vi "Main_v2.vi"() -> ()   [LabVIEW 2018]
uses:
  <userlib>/Gigahertz-Optik/GOMDTR9600/GOMDTR9600.lvlib
panel:
  out "Pulse Begin (ms)":dbl format="%.4f"
  out "Pulse End (ms)":dbl format="%.4f"
  out "Maximum Pulse":cluster{i32[], dbl[]}(graph) caption="Spectrum"
  out "Pulse_Time (µs)":dbl format="%.2f"
  out "Pulse_Energy (V/s)":dbl
  in  "Resolution":u32=10000000
  in  "range100ns":string(combo) caption="Range"
  out "Serial":string
  in  "Sampling Rate":T1(radio)
  in  "range1us":string(combo)="2" caption="Range"
  out "Progress":i32
  in  "ReleaseHandle":bool
  out "Single Measurement":cluster{dbl[], dbl[]}(graph) caption="Spectrum"
  out "State":i32
  in  "measure":bool
  out "Status":string
  # "PULSE ENERGY ANALYZER"
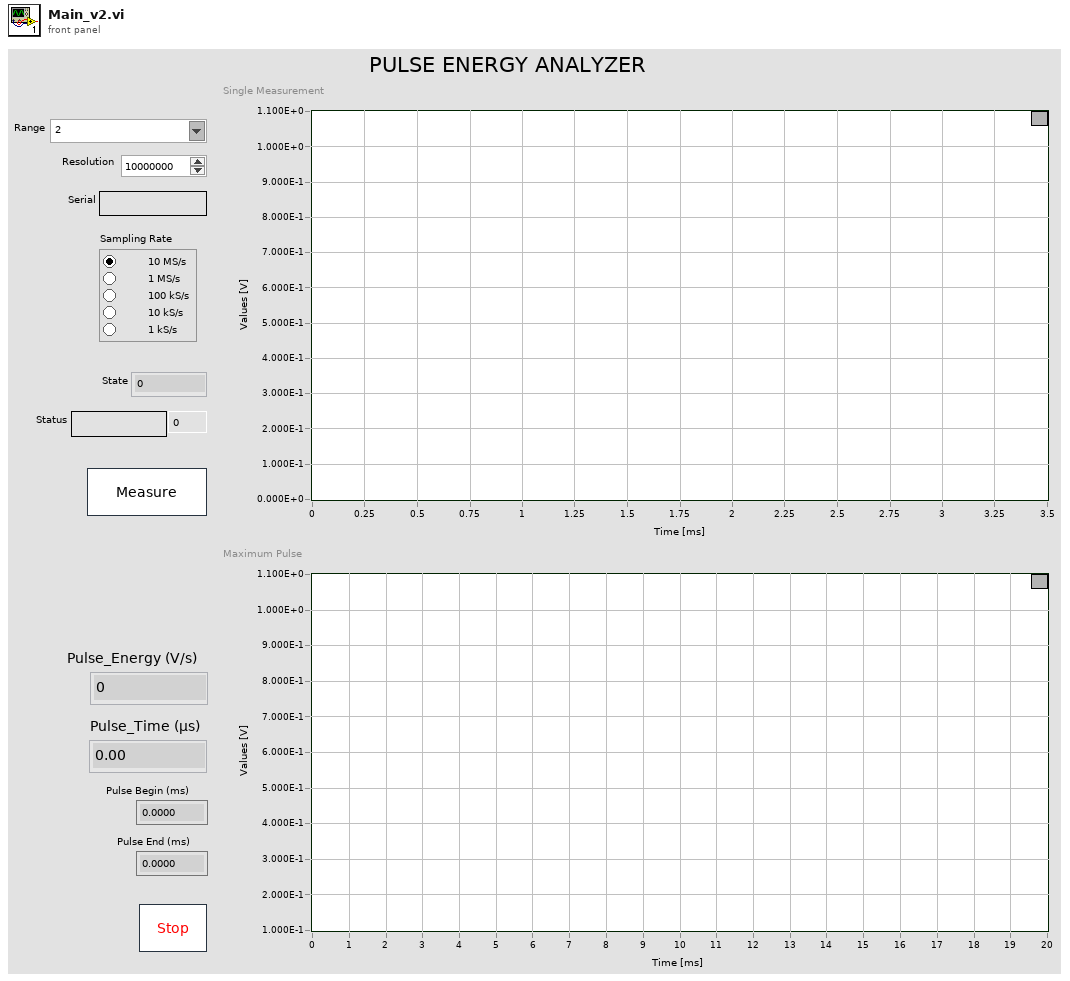
[diagram p1: front panel]
types:
  T1 = enum32{"10MS/s", "1MS/s", "100kS/s", "10kS/s", "1kS/s"}
  T2 = cluster{"address":i32, "mean value":dbl, "min value":dbl, "max value":dbl}[][]
  T3 = enum32{"invalid app kind", "Development System", "Run Time System", "Student Edition", "Embedded LabVIEW", "Evaluation", "Custom"}
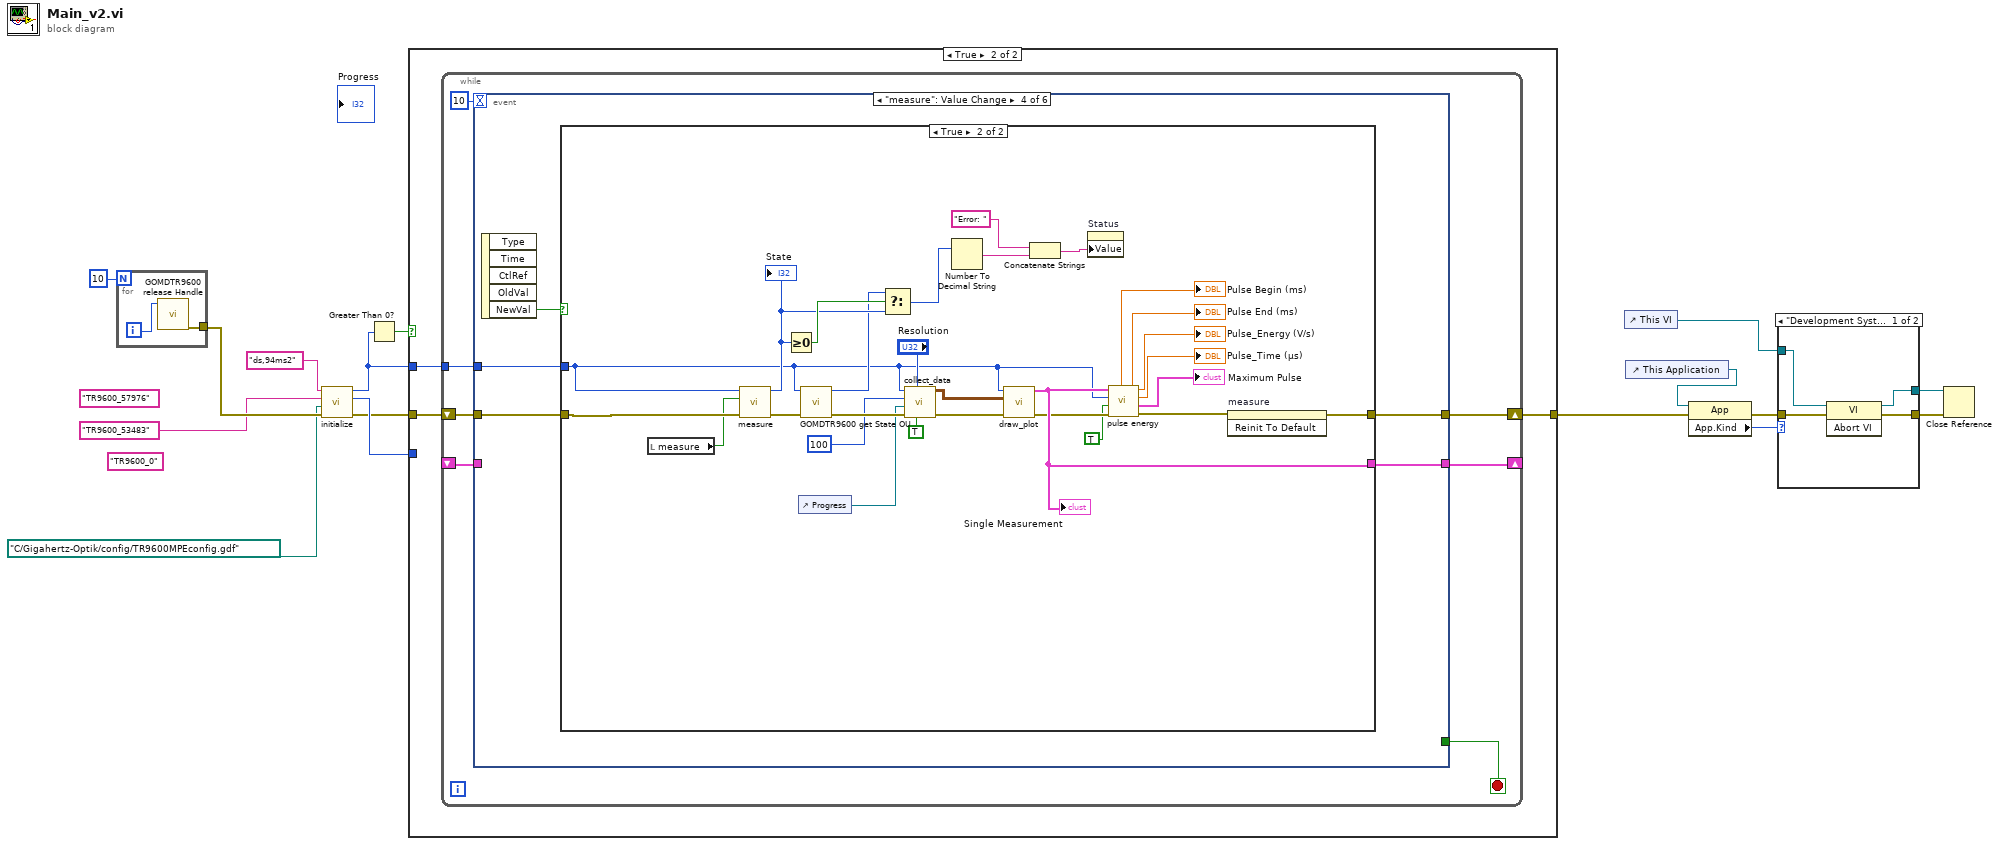
[diagram p0: block diagram]
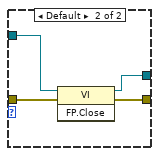
[diagram p2: hidden frame]
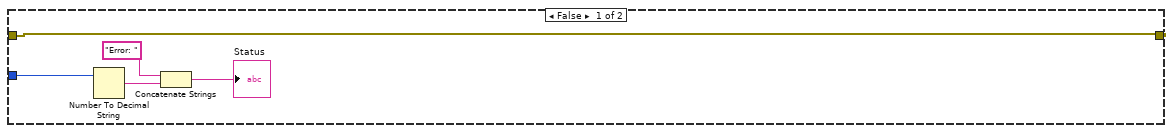
[diagram p3: hidden frame]
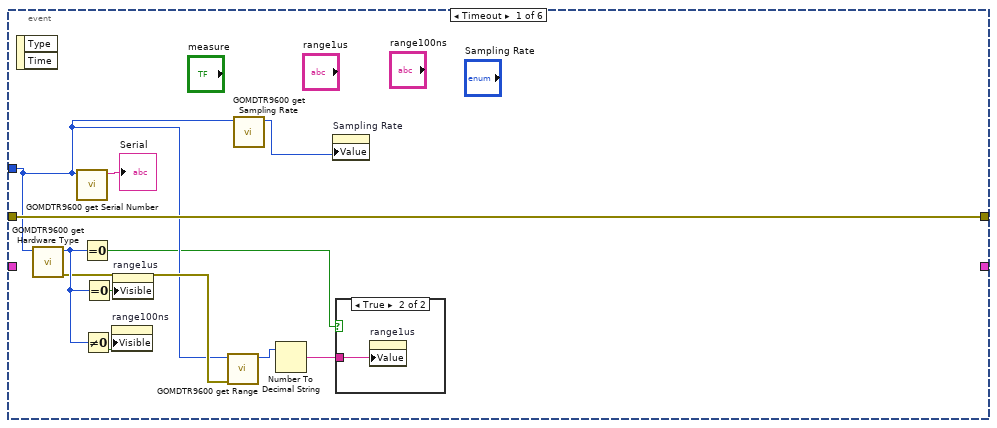
[diagram p4: hidden frame]
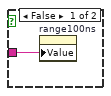
[diagram p5: hidden frame]
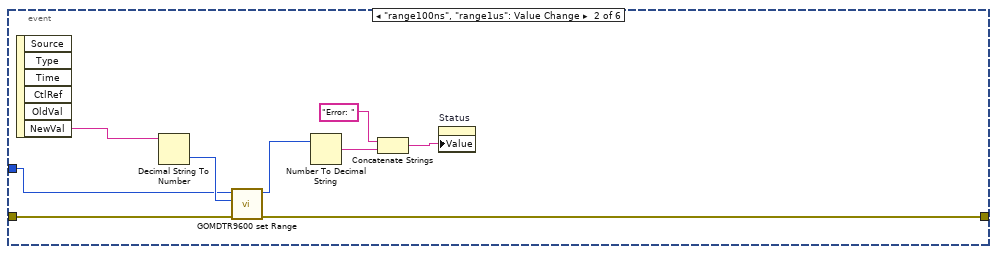
[diagram p6: hidden frame]
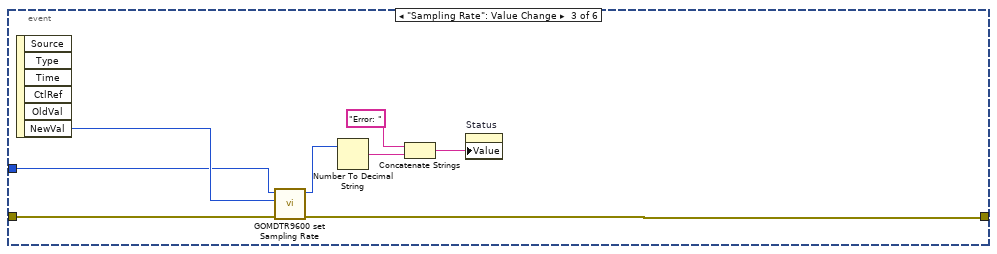
[diagram p7: hidden frame]
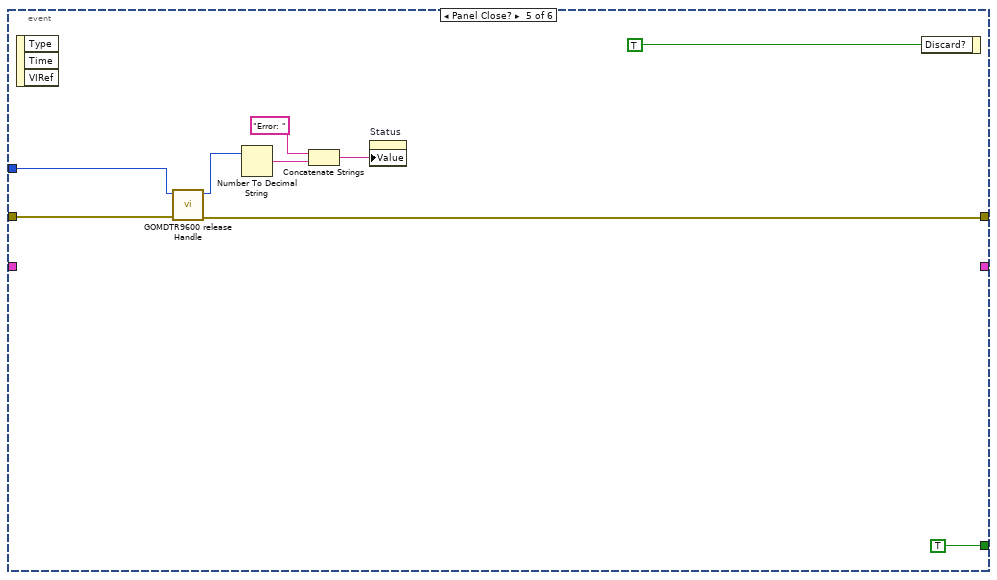
[diagram p9: hidden frame]
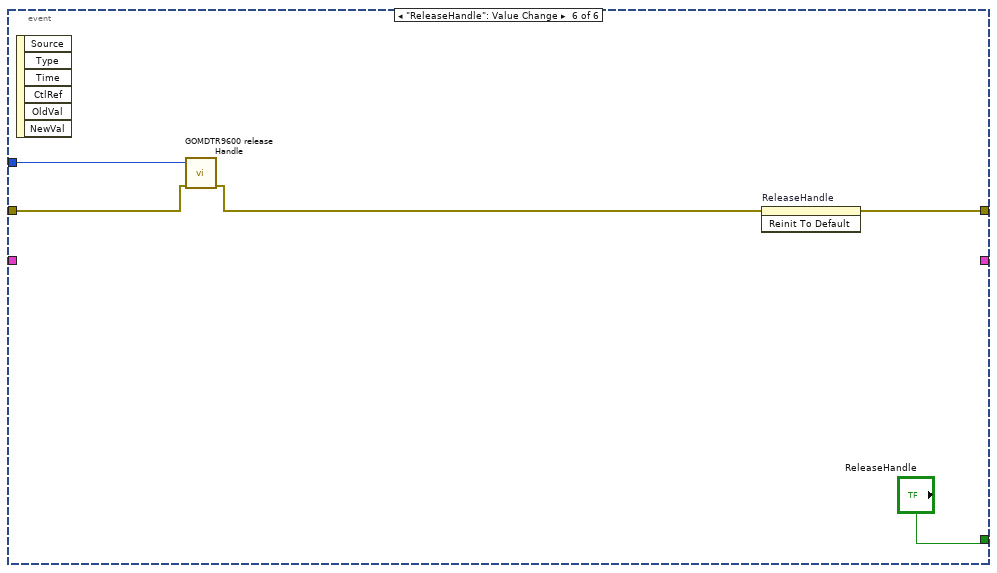
[diagram p10: hidden frame]
diagram:
  (unwired) "TR9600_57976" ("deviceName")
  (unwired) "TR9600_0" ("deviceName")
  n1 = for {
    N: 10 -> [_]
    tunnel: [w17] -> w4
    i -> [w18]
    n2 = call <userlib>:"GOMDTR9600 release Handle.vi"("handle"=w18) -> ("error out"=w17:errorcluster)  [unwired: 9 in, 1 out]
  }
  n3 = call "initialize.vi"("error in (no error)"=w4, "Optometer cfg file"=path "C:/Gigahertz-Optik/config/TR9600MPEconfig.gdf" ("filename"), "deviceName"="TR9600_53483", "password"="ds,94ms2") -> ("error out"=w6:errorcluster, "function return"=w7:i32, "handle"=w3:i32)  [unwired: 5 in]
  n4 = Greater Than 0?(x=w3) -> (x > 0?=w16:bool)
  n5 = case shown="True" w16 {
    tunnel: w3 -> [_ w25]
    tunnel: w6 -> [w19 w26]
    tunnel: w7 -> [w23 _]
    tunnel: [w19 w24] -> w10
    frame False {
      n6 = Number To Decimal String(number=w23) -> (decimal integer string=w21:string)  [unwired: 1 in]
      n7 = Concatenate Strings("Error: ", w21) -> (→"Status":string)
    }
    frame True {
      n8 = while {
        shift-right: [w31] -> w24
        shift-left: w26 -> [w33]
        tunnel: w25 -> [w32]
        shift-right: [w28] -> _
        shift-left: _ -> [w27]
        stop <- w30 stop-if-true
        n9 = event shown="[3] \"measure\": Value Change" {
          selector: _ -> [_ _ _ _ _ _]
          dyn-events: _ -> [_ _ _ _ _ _]
          timeout: 10 -> [_ _ _ _ _ _]
          tunnel: w33 -> [w44 w48 w57 w67 w106 w110]
          tunnel: w32 -> [w35 w49 w58 w66 w105 w111]
          tunnel: [w44 w47 w56 w68 w104 w107] -> w31
          tunnel: [_ _ _ _ TRUE "ReleaseHandle"] -> w30
          tunnel: [_ _ _ w64 _ _] -> w28
          tunnel: w27 -> [_ _ _ _ _ _]
          event Timeout {
            n10 = event-data() -> ()  [unwired: 1 in, 2 out]
            n11 = call <userlib>:"GOMDTR9600 get Hardware Type.vi"("handle"=w35) -> ("error out"=w36:errorcluster, "value"=w39:i32)  [unwired: 8 in, 1 out]
            n12 = call <userlib>:"GOMDTR9600 get Serial Number.vi"("handle"=w35) -> ("value"=→"Serial":string)  [unwired: 8 in, 2 out]
            n13 = Equal To 0?(x=w39) -> (x = 0?=w34:bool)
            n14 = Not Equal To 0?(x=w39) -> (x != 0?=w37:bool)
            n15 = Equal To 0?(x=w39) -> (x = 0?=w38:bool)
            n16 = property on="range100ns" class="CmbBox"("Visible"=w37) -> ()  [unwired: 2 in, 2 out]
            n17 = property on="range1us" class="CmbBox"("Visible"=w38) -> ()  [unwired: 2 in, 2 out]
            n18 = call <userlib>:"GOMDTR9600 get Range.vi"("error in (no error)"=w36, "handle"=w35) -> ("value"=w40:i32)  [unwired: 7 in, 2 out]
            n19 = call <userlib>:"GOMDTR9600 get Sampling Rate.vi"("handle"=w35) -> ("value"=w42:i32)  [unwired: 8 in, 2 out]
            n20 = Number To Decimal String(number=w40) -> (decimal integer string=w41:string)  [unwired: 1 in]
            n21 = property on="Sampling Rate" class="RadioBtnsControl (strict)"("Value"=w42) -> ()  [unwired: 2 in, 2 out]
            n22 = case shown="True" w34 {
              tunnel: w41 -> [w45 w46]
              frame False {
                n23 = property on="range100ns" class="CmbBox"("Value"=w45) -> ()  [unwired: 2 in, 2 out]
              }
              frame True {
                n24 = property on="range1us" class="CmbBox"("Value"=w46) -> ()  [unwired: 2 in, 2 out]
              }
            }
          }
          event "range100ns", "range1us": Value Change {
            n25 = event-data() -> ("NewVal"=w50:string)  [unwired: 1 in, 5 out]
            n26 = Decimal String To Number(string=w50) -> (number=w55:i32)  [unwired: 2 in, 1 out]
            n27 = call <userlib>:"GOMDTR9600 set Range.vi"("error in (no error)"=w48, "value"=w55, "handle"=w49) -> ("error out"=w47:errorcluster, "function return"=w51:i32)  [unwired: 7 in]
            n28 = Number To Decimal String(number=w51) -> (decimal integer string=w52:string)  [unwired: 1 in]
            n29 = Concatenate Strings("Error: ", w52) -> (w54:string)
            n30 = property on="Status" class="Str"("Value"=w54) -> ()  [unwired: 2 in, 2 out]
          }
          event "Sampling Rate": Value Change {
            n31 = event-data() -> ("NewVal"=w59:T1)  [unwired: 1 in, 5 out]
            n32 = call <userlib>:"GOMDTR9600 set Sampling Rate.vi"("error in (no error)"=w57, "value"=w59, "handle"=w58) -> ("error out"=w56:errorcluster, "function return"=w60:i32)  [unwired: 7 in]
            n33 = Number To Decimal String(number=w60) -> (decimal integer string=w61:string)  [unwired: 1 in]
            n34 = Concatenate Strings("Error: ", w61) -> (w63:string)
            n35 = property on="Status" class="Str"("Value"=w63) -> ()  [unwired: 2 in, 2 out]
          }
          event "measure": Value Change {
            n36 = event-data() -> ("NewVal"=w65:bool)  [unwired: 1 in, 4 out]
            n37 = case shown="True" w65 {
              tunnel: [w69 w97] -> w68
              tunnel: w67 -> [w69 w86]
              tunnel: w66 -> [_ w72]
              tunnel: [_ w76] -> w64
              frame False {
              }
              frame True {
                n38 = local read "measure"() -> (w83:bool)
                n39 = call "measure.vi"("error in (no error)"=w86, "Measure"=w83, "handle"=w72) -> ("error out"=w92:errorcluster, "state"=w89:i32)  [unwired: 7 in]
                "State" <- w89
                n40 = Greater Or Equal To 0?(x=w89) -> (x >= 0?=w90:bool)
                n41 = control-ref of="Progress"() -> (w85:refnum<vi>)
                n42 = call <userlib>:"GOMDTR9600 get State OU.vi"("error in (no error)"=w92, "handle"=w72) -> ("error out"=w91:errorcluster, "value"=w88:i32)  [unwired: 7 in, 1 out]
                n43 = Select(t=w88, s=w90, f=w89) -> (s? t:f=w87:i32)
                n44 = call "collect_data.vi"("data?"=TRUE, "Resolution"="Resolution", "error in (no error)"=w91, "progress"=w85, "No. of values"=100, "handle"=w72) -> ("error out"=w96:errorcluster, "Dataset"=w80:T2)  [unwired: 4 in]
                n45 = Number To Decimal String(number=w87) -> (decimal integer string=w93:string)  [unwired: 1 in]
                n46 = call "draw_plot.vi"("error in (no error)"=w96, "Dataset"=w80, "handle"=w72) -> ("error out"=w74:errorcluster, "Plot"=w76:cluster{dbl[], dbl[]})  [unwired: 7 in]
                "Single Measurement" <- w76
                n47 = Concatenate Strings("Error: ", w93) -> (w95:string)
                n48 = property on="Status" class="Str"("Value"=w95) -> ()  [unwired: 2 in, 2 out]
                n49 = call "pulse energy.vi"("error in (no error)"=w74, "Boolean"=TRUE, "handle"=w72, "Spectrum"=w76) -> ("error out"=w75:errorcluster, "MaxPulse"=→"Maximum Pulse":cluster{i32[], dbl[]}, "Pulse_time"=→"Pulse_Time (µs)":dbl, "PulseEnergy"=→"Pulse_Energy (V/s)":dbl, "Pulse End"=→"Pulse End (ms)":dbl, "Pulse Begin"=→"Pulse Begin (ms)":dbl)  [unwired: 2 in]
                n50 = invoke on="measure" class="Bool (strict)" method="Reinit To Default"(error in=w75) -> (error out=w97:errorcluster)  [unwired: 2 in, 2 out]
              }
            }
          }
          event Panel Close? {
            n51 = event-data() -> ()  [unwired: 1 in, 3 out]
            n52 = call <userlib>:"GOMDTR9600 release Handle.vi"("error in (no error)"=w106, "handle"=w105) -> ("error out"=w104:errorcluster, "function return"=w99:i32)  [unwired: 8 in]
            n53 = Number To Decimal String(number=w99) -> (decimal integer string=w100:string)  [unwired: 1 in]
            n54 = Concatenate Strings("Error: ", w100) -> (w102:string)
            n55 = property on="Status" class="Str"("Value"=w102) -> ()  [unwired: 2 in, 2 out]
            n56 = event-data("Discard?"=TRUE) -> ()  [unwired: 1 in, 1 out]
          }
          event "ReleaseHandle": Value Change {
            n57 = event-data() -> ()  [unwired: 1 in, 6 out]
            n58 = call <userlib>:"GOMDTR9600 release Handle.vi"("error in (no error)"=w110, "handle"=w111) -> ("error out"=w108:errorcluster)  [unwired: 8 in, 1 out]
            n59 = invoke on="ReleaseHandle" class="Bool (strict)" method="Reinit To Default"(error in=w108) -> (error out=w107:errorcluster)  [unwired: 2 in, 2 out]
          }
        }
      }
    }
  }
  n60 = control-ref of="This VI"() -> (w11:refnum<vi>)
  n61 = control-ref of="This Application"() -> (w9:refnum<vi>)
  n62 = property class="App"(reference=w9, error in=w10) -> (error out=w14:errorcluster, "App.Kind"=w15:T3)  [unwired: 1 out]
  n63 = case shown="\"Development System\"" w15 {
    tunnel: w14 -> [w115 w119]
    tunnel: [w113 w117] -> w12
    tunnel: w11 -> [w112 w118]
    tunnel: [w114 w116] -> w13
    frame "Development System" {
      n64 = invoke class="VI" method="Abort VI"(reference=w112, error in=w115) -> (reference out=w114:refnum<vi>, error out=w113:errorcluster)  [unwired: 1 in, 1 out]
    }
    frame Default {
      n65 = invoke class="VI" method="FP.Close"(reference=w118, error in=w119) -> (reference out=w116:refnum<vi>, error out=w117:errorcluster)  [unwired: 1 in, 1 out]
    }
  }
  n66 = Close Reference(reference=w13, error in (no error)=w12) -> ()  [unwired: 1 out]
